vi "quiz3.5.vi"() -> ()   [LabVIEW 2017]
panel:
  out "Tab Control 2":enum32{"Login", "Menu", "Add", "delete"}(tab)
  in  "Ingresar 2":bool
  in  "Contraseña 2":string
  in  "Usuario 2":string
  in  "Delete Button 2":bool
  in  "Add Button 2":bool
  in  "Home Button 2":bool
  out "Cusuario 2":string
  in  "Previous Button 3":bool
  in  "AddContraseña 2":string
  in  "AddUsuario 2":string
  in  "Agregar 2":bool
  out "Agregado 2":bool
  in  "Cancel Button 2":bool
  in  "DeleteUsuario 2":string
  in  "Previous Button 4":bool
  out "text 2":string caption="Usuarios Activos"
  out "Tab Control":enum32{"Login", "Menu", "Add", "delete"}(tab)
  in  "Ingresar":bool
  in  "Contraseña":string
  in  "Usuario":string
  in  "Delete Button":bool
  in  "Add Button":bool
  in  "Home Button":bool
  out "Cusuario":string
  in  "Previous Button":bool
  in  "AddContraseña":string
  in  "AddUsuario":string
  in  "Agregar":bool
  out "Agregado":bool
  in  "Cancel Button":bool
  in  "DeleteUsuario":string
  in  "Previous Button 2":bool
  out "text":string caption="Usuarios Activos"
  # "USTED INGRESO CON EL USUARIO"
  # "USTED INGRESO CON EL USUARIO"
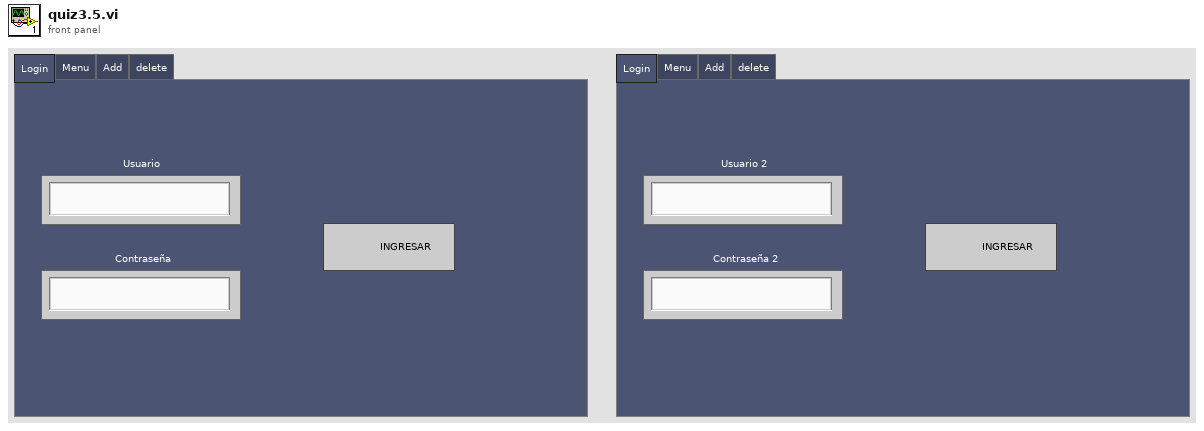
[diagram p1: front panel]
types:
  T1 = enum16{"open", "replace", "create", "open or create", "replace or create", "replace or create with confirmation"}
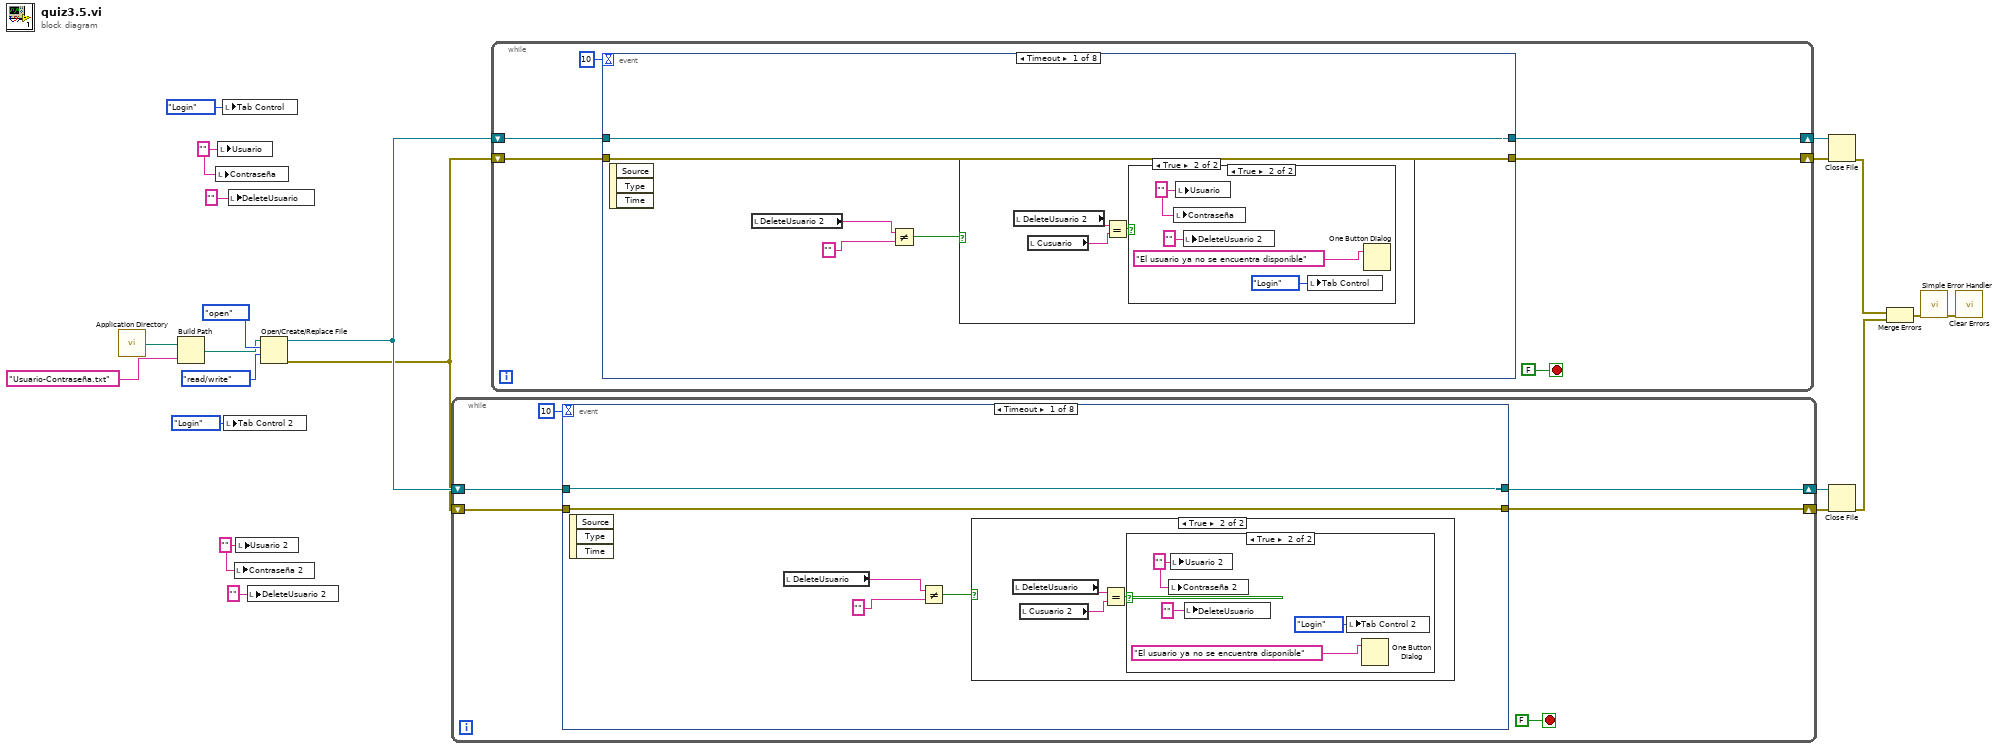
[diagram p0: block diagram]
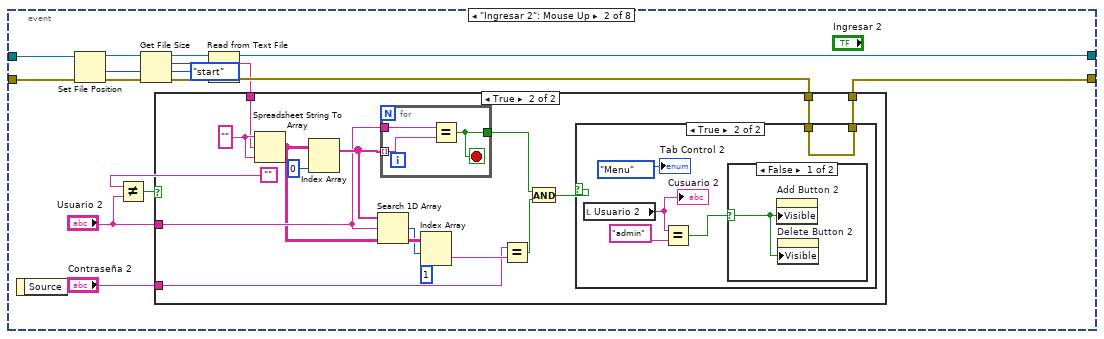
[diagram p4: hidden frame]
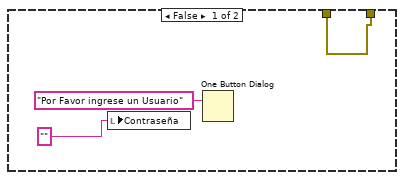
[diagram p5: hidden frame]
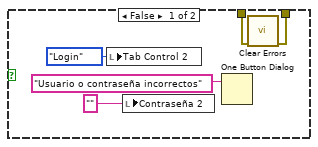
[diagram p6: hidden frame]
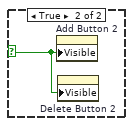
[diagram p7: hidden frame]
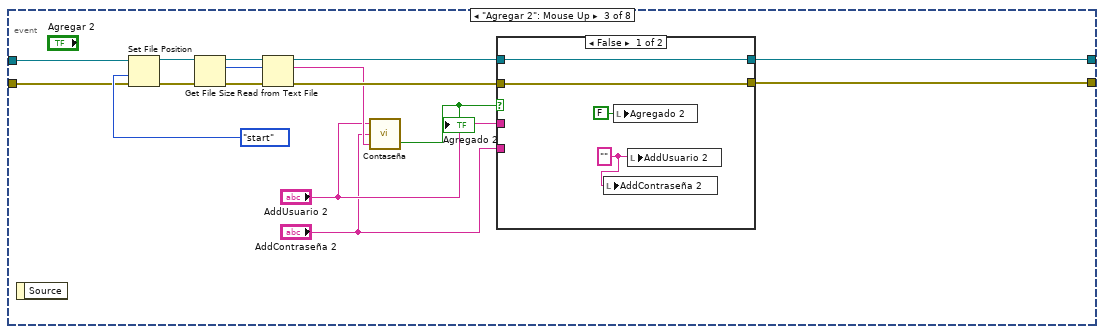
[diagram p8: hidden frame]
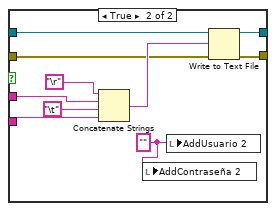
[diagram p9: hidden frame]
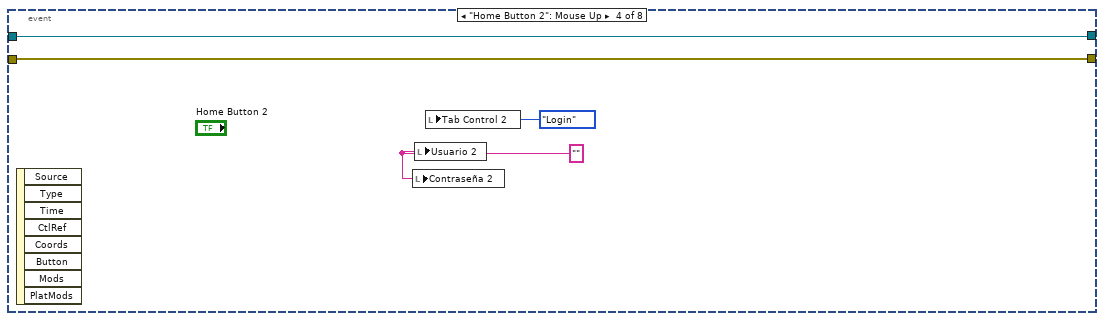
[diagram p10: hidden frame]
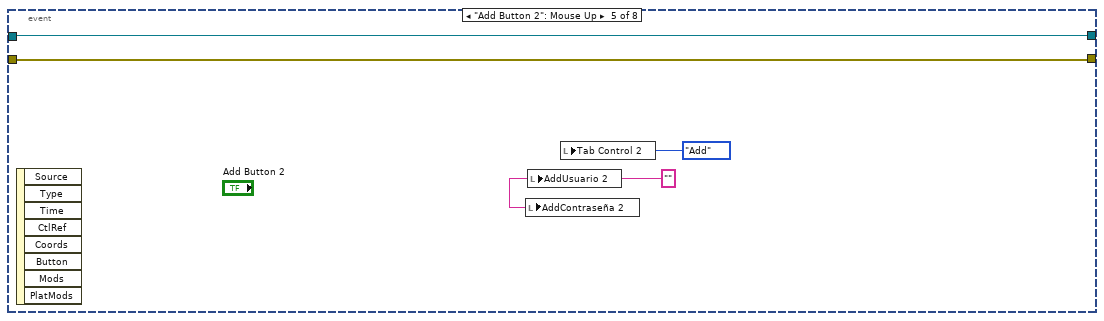
[diagram p11: hidden frame]
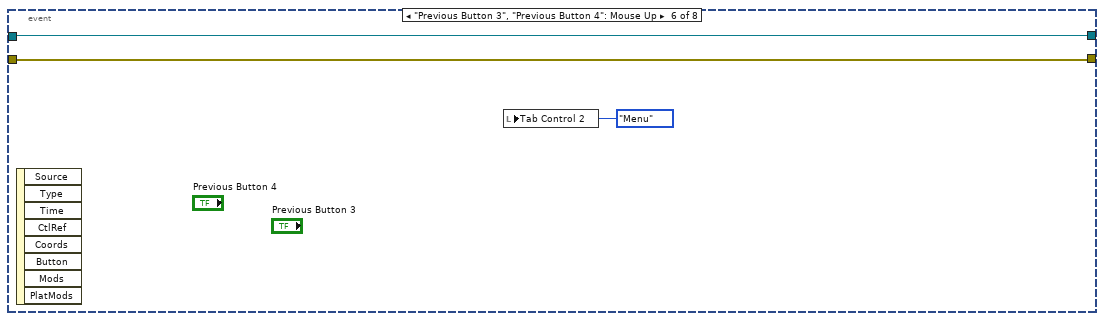
[diagram p12: hidden frame]
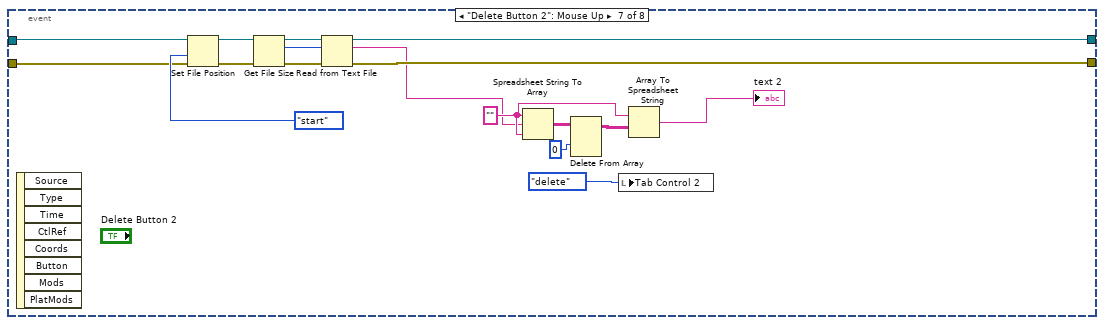
[diagram p13: hidden frame]
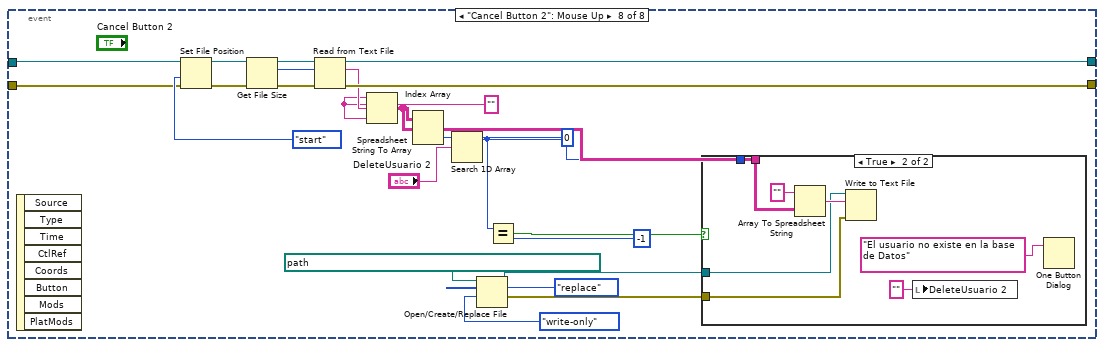
[diagram p14: hidden frame]
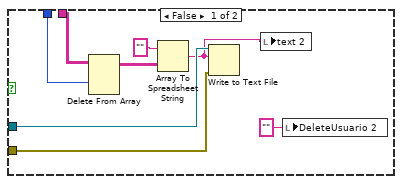
[diagram p15: hidden frame]
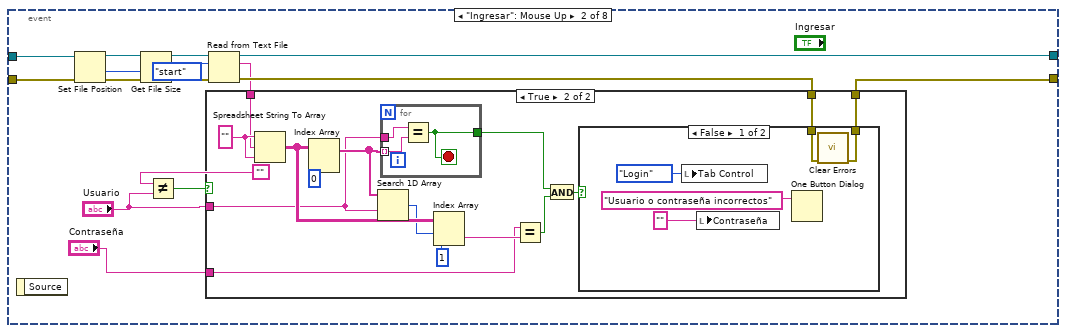
[diagram p18: hidden frame]
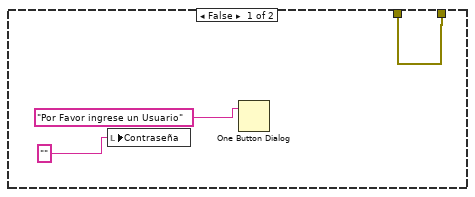
[diagram p19: hidden frame]
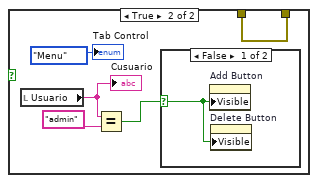
[diagram p20: hidden frame]
diagram:
  w2 = "" ("Usuario")
  w14 = "" ("Usuario")
  n1 = call <vilib>:"Application Directory.vi"() -> ("Application Directory"=w21:path)
  n2 = Build Path(base path=w21, name or relative path="Usuario-Contraseña.txt") -> (appended path=w15:path)
  n3 = local write "Contraseña"(w14) -> ()
  n4 = local write "Usuario"(w14) -> ()
  n5 = local write "Tab Control"(enum32{"Login", "Menu", "Add", "delete"}."Login" ("Tab Control")) -> ()
  n6 = local write "Tab Control 2"(enum32{"Login", "Menu", "Add", "delete"}."Login" ("Tab Control")) -> ()
  n7 = local write "DeleteUsuario"("" ("DeleteUsuario 2")) -> ()
  n8 = local write "Contraseña 2"(w2) -> ()
  n9 = local write "Usuario 2"(w2) -> ()
  n10 = local write "DeleteUsuario 2"("" ("DeleteUsuario 2")) -> ()
  n11 = Open/Create/Replace File(file path (use dialog)=w15, operation (0:open)=T1."open", access (0:read/write)=enum16{"read/write", "read-only", "write-only"}."read/write") -> (refnum out=w5:refnum<file>, error out=w3:errorcluster)  [unwired: 3 in, 1 out]
  n12 = while {
    shift-right: [w24] -> w6
    shift-left: w5 -> [w25]
    shift-right: [w23] -> w7
    shift-left: w3 -> [w26]
    stop <- FALSE stop-if-true
    n13 = event shown="[0] Timeout" {
      selector: _ -> [_ _ _ _ _ _ _ _]
      dyn-events: _ -> [_ _ _ _ _ _ _ _]
      timeout: 10 -> [_ _ _ _ _ _ _ _]
      tunnel: w26 -> [w31 w55 w92 w120 w125 w128 w137 w164]
      tunnel: [w32 w50 w104 w121 w126 w129 w138 w160] -> w24
      tunnel: [w31 w47 w103 w120 w125 w128 w136 w159] -> w23
      tunnel: w25 -> [w32 w49 w93 w121 w126 w129 w139 w163]
      event Timeout {
        n14 = event-data() -> ()  [unwired: 1 in, 3 out]
        n15 = local read "DeleteUsuario"() -> (w29:string)
        n16 = Not Equal?(x=w29, y="" ("DeleteUsuario 2")) -> (x != y?=w30:bool)
        n17 = case shown="True" w30 {
          frame False {
          }
          frame True {
            n18 = local read "DeleteUsuario"() -> (w34:string)
            n19 = local read "Cusuario 2"() -> (w33:string)
            n20 = Equal?(x=w34, y=w33) -> (x = y?=w35:bool)
            n21 = case shown="True" w35 {
              frame False {
              }
              frame True {
                w36 = "" ("Usuario")
                n22 = local write "Contraseña 2"(w36) -> ()
                n23 = local write "Usuario 2"(w36) -> ()
                n24 = local write "DeleteUsuario"("" ("DeleteUsuario 2")) -> ()
                n25 = local write "Tab Control 2"(enum32{"Login", "Menu", "Add", "delete"}."Login" ("Tab Control")) -> ()
                n26 = One Button Dialog(message="El usuario ya no se encuentra disponible") -> ()  [unwired: 1 in, 1 out]
              }
            }
          }
        }
      }
      event "Ingresar 2": Mouse Up {
        n27 = event-data() -> ()  [unwired: 1 in, 1 out]
        n28 = Set File Position(refnum=w49, from (0:start)=enum16{"start", "end", "current"}."start", error in=w55) -> (refnum out=w53:refnum<file>, error out=w54:errorcluster)  [unwired: 1 in]
        n29 = Not Equal?(x="", y="Usuario 2") -> (x != y?=w41:bool)
        n30 = Get File Size(file=w53, error in=w54) -> (refnum out=w45:refnum<file>, size (in bytes)=w52:i64, 0:w51:errorcluster)
        n31 = Read from Text File(file (use dialog)=w45, count=w52, error in=w51) -> (refnum out=w50:refnum<file>, text=w44:string, error out=w48:errorcluster)  [unwired: 1 in, 1 out]
        n32 = case shown="True" w41 {
          tunnel: w48 -> [w58 w73]
          tunnel: [w58 w72] -> w47
          tunnel: w44 -> [_ w69]
          tunnel: "Usuario 2" -> [_ w66]
          tunnel: "Contraseña 2" -> [_ w59]
          frame False {
            n33 = local write "Contraseña"("" ("Usuario")) -> ()
            n34 = One Button Dialog(message="Por Favor ingrese un Usuario") -> ()  [unwired: 1 in, 1 out]
          }
          frame True {
            w70 = "" ("format string")
            n35 = Spreadsheet String To Array(format string=w70, spreadsheet string=w69, array type (2D Dbl)=w70) -> (array=w65:string[][])  [unwired: 1 in]
            n36 = Index Array(array=w65, index (col)=0 ("index")) -> (element=w67:string[])  [unwired: 1 in]
            n37 = Search 1D Array(1D array=w67, element=w66) -> (index of element=w62:i32)  [unwired: 1 in]
            n38 = for {
              tunnel: w66 -> [w76]
              tunnel: [w75] -> w68
              tunnel: w67 -> [w74] mode=indexing
              stop <- w75 stop-if-true
              n39 = Equal?(x=w76, y=w74) -> (x = y?=w75:bool)
            }
            n40 = Index Array(array=w65, index (row)=w62, index (col)=1 ("index")) -> (element=w60:string)
            n41 = Equal?(x=w59, y=w60) -> (x = y?=w64:bool)
            n42 = And(x=w68, y=w64) -> (x .and. y?=w71:bool)
            n43 = case shown="True" w71 {
              tunnel: [w79 w86] -> w72
              tunnel: w73 -> [w78 w86]
              frame False {
                n44 = local write "Tab Control 2"(enum32{"Login", "Menu", "Add", "delete"}."Login" ("Tab Control")) -> ()
                n45 = local write "Contraseña 2"("" ("Usuario")) -> ()
                n46 = One Button Dialog(message="Usuario o contraseña incorrectos") -> ()  [unwired: 1 in, 1 out]
                n47 = call <vilib>:"Clear Errors.vi"("error in (no error)"=w78) -> ("error out"=w79:errorcluster)  [unwired: 5 in, 1 out]
              }
              frame True {
                n48 = local read "Usuario 2"() -> (w84:string)
                "Cusuario 2" <- w84
                n49 = Equal?(x=w84, y="admin") -> (x = y?=w85:bool)
                n50 = case shown="False" w85 {
                  selector: w85 -> [w87 w88]
                  frame False {
                    n51 = property on="Add Button 2" class="Bool (strict)"("Visible"=w87) -> ()  [unwired: 2 in, 2 out]
                    n52 = property on="Delete Button 2" class="Bool (strict)"("Visible"=w87) -> ()  [unwired: 2 in, 2 out]
                  }
                  frame True {
                    n53 = property on="Add Button 2" class="Bool (strict)"("Visible"=w88) -> ()  [unwired: 2 in, 2 out]
                    n54 = property on="Delete Button 2" class="Bool (strict)"("Visible"=w88) -> ()  [unwired: 2 in, 2 out]
                  }
                }
                "Tab Control 2" <- enum32{"Login", "Menu", "Add", "delete"}."Menu" ("Tab Control")
              }
            }
          }
        }
      }
      event "Agregar 2": Mouse Up {
        n55 = event-data() -> ()  [unwired: 1 in, 1 out]
        n56 = Set File Position(refnum=w93, from (0:start)=enum16{"start", "end", "current"}."start", error in=w92) -> (refnum out=w100:refnum<file>, error out=w101:errorcluster)  [unwired: 1 in]
        n57 = Get File Size(file=w100, error in=w101) -> (refnum out=w97:refnum<file>, size (in bytes)=w99:i64, 0:w98:errorcluster)
        n58 = Read from Text File(file (use dialog)=w97, count=w99, error in=w98) -> (refnum out=w95:refnum<file>, text=w91:string, error out=w94:errorcluster)  [unwired: 1 in, 1 out]
        n59 = call "Contaseña.vi"("spreadsheet string"=w91, "AddContraseña"="AddContraseña 2", "addUsuario"="AddUsuario 2") -> ("result"=w102:bool)  [unwired: 1 out]
        "Agregado 2" <- w102
        n60 = case shown="False" w102 {
          tunnel: [w108 w118] -> w104
          tunnel: [w107 w117] -> w103
          tunnel: w95 -> [w108 w113]
          tunnel: w94 -> [w107 w112]
          tunnel: "AddUsuario 2" -> [_ w111]
          tunnel: "AddContraseña 2" -> [_ w110]
          frame False {
            w106 = "" ("Usuario")
            n61 = local write "AddContraseña 2"(w106) -> ()
            n62 = local write "Agregado 2"(FALSE ("Agregado")) -> ()
            n63 = local write "AddUsuario 2"(w106) -> ()
          }
          frame True {
            w109 = "" ("Usuario")
            n64 = Concatenate Strings("\r", w111, "\t", w110) -> (w116:string)
            n65 = local write "AddContraseña 2"(w109) -> ()
            n66 = local write "AddUsuario 2"(w109) -> ()
            n67 = Write to Text File(file (use dialog)=w113, text=w116, error in=w112) -> (refnum out=w118:refnum<file>, error out=w117:errorcluster)  [unwired: 1 in, 1 out]
          }
        }
      }
      event "Home Button 2": Mouse Up {
        w122 = "" ("Usuario")
        n68 = event-data() -> ()  [unwired: 1 in, 8 out]
        n69 = local write "Contraseña 2"(w122) -> ()
        n70 = local write "Usuario 2"(w122) -> ()
        n71 = local write "Tab Control 2"(enum32{"Login", "Menu", "Add", "delete"}."Login" ("Tab Control")) -> ()
      }
      event "Add Button 2": Mouse Up {
        w123 = "" ("Usuario")
        n72 = event-data() -> ()  [unwired: 1 in, 8 out]
        n73 = local write "AddContraseña 2"(w123) -> ()
        n74 = local write "AddUsuario 2"(w123) -> ()
        n75 = local write "Tab Control 2"(enum32{"Login", "Menu", "Add", "delete"}."Add" ("Tab Control")) -> ()
      }
      event "Previous Button 3", "Previous Button 4": Mouse Up {
        n76 = event-data() -> ()  [unwired: 1 in, 8 out]
        n77 = local write "Tab Control 2"(enum32{"Login", "Menu", "Add", "delete"}."Menu" ("Tab Control")) -> ()
      }
      event "Delete Button 2": Mouse Up {
        w135 = "" ("format string")
        n78 = event-data() -> ()  [unwired: 1 in, 8 out]
        n79 = Set File Position(refnum=w139, from (0:start)=enum16{"start", "end", "current"}."start", error in=w137) -> (refnum out=w144:refnum<file>, error out=w145:errorcluster)  [unwired: 1 in]
        n80 = Get File Size(file=w144, error in=w145) -> (refnum out=w141:refnum<file>, size (in bytes)=w143:i64, 0:w142:errorcluster)
        n81 = Read from Text File(file (use dialog)=w141, count=w143, error in=w142) -> (refnum out=w138:refnum<file>, text=w131:string, error out=w136:errorcluster)  [unwired: 1 in, 1 out]
        n82 = Spreadsheet String To Array(format string=w135, spreadsheet string=w131, array type (2D Dbl)=w135) -> (array=w133:string[][])  [unwired: 1 in]
        n83 = Delete From Array(array=w133, index (row)=0) -> (array with subset deleted=w132:string[][])  [unwired: 2 in, 1 out]
        n84 = local write "Tab Control 2"(enum32{"Login", "Menu", "Add", "delete"}."delete" ("Tab Control")) -> ()
        n85 = Array To Spreadsheet String(array=w132, 3:w135) -> (spreadsheet string=→"text 2":string)  [unwired: 1 in]
      }
      event "Cancel Button 2": Mouse Up {
        w156 = "" ("format string")
        n86 = event-data() -> ()  [unwired: 1 in, 8 out]
        n87 = Set File Position(refnum=w163, from (0:start)=enum16{"start", "end", "current"}."start", error in=w164) -> (refnum out=w169:refnum<file>, error out=w170:errorcluster)  [unwired: 1 in]
        n88 = Get File Size(file=w169, error in=w170) -> (refnum out=w166:refnum<file>, size (in bytes)=w168:i64, 0:w167:errorcluster)
        n89 = Read from Text File(file (use dialog)=w166, count=w168, error in=w167) -> (refnum out=w160:refnum<file>, text=w157:string, error out=w159:errorcluster)  [unwired: 1 in, 1 out]
        n90 = Spreadsheet String To Array(format string=w156, spreadsheet string=w157, array type (2D Dbl)=w156) -> (array=w152:string[][])  [unwired: 1 in]
        n91 = Index Array(array=w152, index (col)=0 ("disabled index (col)")) -> (element=w154:string[])  [unwired: 1 in]
        n92 = Search 1D Array(1D array=w154, element="DeleteUsuario 2") -> (index of element=w148:i32)  [unwired: 1 in]
        n93 = Open/Create/Replace File(file path (use dialog)=path "D:/2019-1/Programacion 2/quiz 3/Usuario-Contraseña.txt", operation (0:open)=T1."replace", access (0:read/write)=enum16{"read/write", "read-only", "write-only"}."write-only") -> (refnum out=w151:refnum<file>, error out=w150:errorcluster)  [unwired: 3 in, 1 out]
        n94 = Equal?(x=w148, y=-1) -> (x = y?=w149:bool)
        n95 = case shown="True" w149 {
          tunnel: w152 -> [w178 w181]
          tunnel: w148 -> [w177 _]
          tunnel: w151 -> [w175 w180]
          tunnel: w150 -> [w174 w179]
          frame False {
            n96 = Delete From Array(array=w178, index (row)=w177) -> (array with subset deleted=w176:string[][])  [unwired: 2 in, 1 out]
            n97 = Array To Spreadsheet String(array=w176, 3:"" ("format string")) -> (spreadsheet string=w172:string)  [unwired: 1 in]
            n98 = Write to Text File(file (use dialog)=w175, text=w172, error in=w174) -> ()  [unwired: 1 in, 3 out]
            n99 = local write "text 2"(w172) -> ()
            n100 = local write "DeleteUsuario 2"("" ("DeleteUsuario 2")) -> ()
          }
          frame True {
            n101 = Array To Spreadsheet String(array=w181, 3:"" ("format string")) -> (spreadsheet string=w183:string)  [unwired: 1 in]
            n102 = Write to Text File(file (use dialog)=w180, text=w183, error in=w179) -> ()  [unwired: 1 in, 3 out]
            n103 = local write "DeleteUsuario 2"("" ("DeleteUsuario 2")) -> ()
            n104 = One Button Dialog(message="El usuario no existe en la base de Datos") -> ()  [unwired: 1 in, 1 out]
          }
        }
      }
    }
  }
  n105 = while {
    shift-right: [w188] -> w11
    shift-left: w5 -> [w189]
    shift-right: [w187] -> w16
    shift-left: w3 -> [w190]
    stop <- FALSE stop-if-true
    n106 = event shown="[0] Timeout" {
      selector: _ -> [_ _ _ _ _ _ _ _]
      dyn-events: _ -> [_ _ _ _ _ _ _ _]
      timeout: 10 -> [_ _ _ _ _ _ _ _]
      tunnel: w190 -> [w195 w219 w257 w284 w289 w292 w301 w328]
      tunnel: [w196 w214 w268 w285 w290 w293 w302 w324] -> w188
      tunnel: [w195 w211 w253 w284 w289 w292 w300 w323] -> w187
      tunnel: w189 -> [w196 w213 w258 w285 w290 w293 w303 w327]
      event Timeout {
        n107 = event-data() -> ()  [unwired: 1 in, 3 out]
        n108 = local read "DeleteUsuario 2"() -> (w193:string)
        n109 = Not Equal?(x=w193, y="" ("DeleteUsuario 2")) -> (x != y?=w192:bool)
        n110 = case shown="True" w192 {
          frame False {
          }
          frame True {
            n111 = local read "DeleteUsuario 2"() -> (w197:string)
            n112 = local read "Cusuario"() -> (w198:string)
            n113 = Equal?(x=w197, y=w198) -> (x = y?=w199:bool)
            n114 = case shown="True" w199 {
              frame False {
              }
              frame True {
                w200 = "" ("Usuario")
                n115 = local write "Contraseña"(w200) -> ()
                n116 = local write "Usuario"(w200) -> ()
                n117 = local write "DeleteUsuario 2"("" ("DeleteUsuario 2")) -> ()
                n118 = local write "Tab Control"(enum32{"Login", "Menu", "Add", "delete"}."Login" ("Tab Control")) -> ()
                n119 = One Button Dialog(message="El usuario ya no se encuentra disponible") -> ()  [unwired: 1 in, 1 out]
              }
            }
          }
        }
      }
      event "Ingresar": Mouse Up {
        n120 = event-data() -> ()  [unwired: 1 in, 1 out]
        n121 = Set File Position(refnum=w213, from (0:start)=enum16{"start", "end", "current"}."start", error in=w219) -> (refnum out=w217:refnum<file>, error out=w218:errorcluster)  [unwired: 1 in]
        n122 = Get File Size(file=w217, error in=w218) -> (refnum out=w209:refnum<file>, size (in bytes)=w216:i64, 0:w215:errorcluster)
        n123 = Not Equal?(x="", y="Usuario") -> (x != y?=w206:bool)
        n124 = Read from Text File(file (use dialog)=w209, count=w216, error in=w215) -> (refnum out=w214:refnum<file>, text=w208:string, error out=w212:errorcluster)  [unwired: 1 in, 1 out]
        n125 = case shown="True" w206 {
          tunnel: w212 -> [w222 w237]
          tunnel: [w222 w236] -> w211
          tunnel: w208 -> [_ w233]
          tunnel: "Usuario" -> [_ w224]
          tunnel: "Contraseña" -> [_ w223]
          frame False {
            n126 = local write "Contraseña"("" ("Usuario")) -> ()
            n127 = One Button Dialog(message="Por Favor ingrese un Usuario") -> ()  [unwired: 1 in, 1 out]
          }
          frame True {
            w234 = "" ("format string")
            n128 = Spreadsheet String To Array(format string=w234, spreadsheet string=w233, array type (2D Dbl)=w234) -> (array=w230:string[][])  [unwired: 1 in]
            n129 = Index Array(array=w230, index (col)=0 ("index")) -> (element=w231:string[])  [unwired: 1 in]
            n130 = Search 1D Array(1D array=w231, element=w224) -> (index of element=w227:i32)  [unwired: 1 in]
            n131 = for {
              tunnel: [w240] -> w232
              tunnel: w231 -> [w239] mode=indexing
              tunnel: w224 -> [w238]
              stop <- w240 stop-if-true
              n132 = Equal?(x=w238, y=w239) -> (x = y?=w240:bool)
            }
            n133 = Index Array(array=w230, index (row)=w227, index (col)=1 ("index")) -> (element=w225:string)
            n134 = Equal?(x=w223, y=w225) -> (x = y?=w229:bool)
            n135 = And(x=w232, y=w229) -> (x .and. y?=w235:bool)
            n136 = case shown="False" w235 {
              tunnel: [w243 w250] -> w236
              tunnel: w237 -> [w242 w250]
              frame False {
                n137 = local write "Tab Control"(enum32{"Login", "Menu", "Add", "delete"}."Login" ("Tab Control")) -> ()
                n138 = local write "Contraseña"("" ("Usuario")) -> ()
                n139 = One Button Dialog(message="Usuario o contraseña incorrectos") -> ()  [unwired: 1 in, 1 out]
                n140 = call <vilib>:"Clear Errors.vi"("error in (no error)"=w242) -> ("error out"=w243:errorcluster)  [unwired: 5 in, 1 out]
              }
              frame True {
                n141 = local read "Usuario"() -> (w248:string)
                "Cusuario" <- w248
                n142 = Equal?(x=w248, y="admin") -> (x = y?=w249:bool)
                n143 = case shown="False" w249 {
                  selector: w249 -> [w251 w252]
                  frame False {
                    n144 = property on="Add Button" class="Bool (strict)"("Visible"=w251) -> ()  [unwired: 2 in, 2 out]
                    n145 = property on="Delete Button" class="Bool (strict)"("Visible"=w251) -> ()  [unwired: 2 in, 2 out]
                  }
                  frame True {
                    n146 = property on="Add Button" class="Bool (strict)"("Visible"=w252) -> ()  [unwired: 2 in, 2 out]
                    n147 = property on="Delete Button" class="Bool (strict)"("Visible"=w252) -> ()  [unwired: 2 in, 2 out]
                  }
                }
                "Tab Control" <- enum32{"Login", "Menu", "Add", "delete"}."Menu" ("Tab Control")
              }
            }
          }
        }
      }
      event "Agregar": Mouse Up {
        n148 = event-data() -> ()  [unwired: 1 in, 1 out]
        n149 = Set File Position(refnum=w258, from (0:start)=enum16{"start", "end", "current"}."start", error in=w257) -> (refnum out=w265:refnum<file>, error out=w266:errorcluster)  [unwired: 1 in]
        n150 = Get File Size(file=w265, error in=w266) -> (refnum out=w262:refnum<file>, size (in bytes)=w264:i64, 0:w263:errorcluster)
        n151 = Read from Text File(file (use dialog)=w262, count=w264, error in=w263) -> (refnum out=w260:refnum<file>, text=w256:string, error out=w259:errorcluster)  [unwired: 1 in, 1 out]
        n152 = call "Contaseña.vi"("spreadsheet string"=w256, "AddContraseña"="AddContraseña", "addUsuario"="AddUsuario") -> ("result"=w267:bool)  [unwired: 1 out]
        "Agregado" <- w267
        n153 = case shown="False" w267 {
          tunnel: [w272 w282] -> w268
          tunnel: [w271 w281] -> w253
          tunnel: w260 -> [w272 w277]
          tunnel: w259 -> [w271 w276]
          tunnel: "AddUsuario" -> [_ w275]
          tunnel: "AddContraseña" -> [_ w274]
          frame False {
            w270 = "" ("Usuario")
            n154 = local write "AddContraseña"(w270) -> ()
            n155 = local write "Agregado"(FALSE ("Agregado")) -> ()
            n156 = local write "AddUsuario"(w270) -> ()
          }
          frame True {
            w273 = "" ("Usuario")
            n157 = Concatenate Strings("\r", w275, "\t", w274) -> (w280:string)
            n158 = local write "AddContraseña"(w273) -> ()
            n159 = local write "AddUsuario"(w273) -> ()
            n160 = Write to Text File(file (use dialog)=w277, text=w280, error in=w276) -> (refnum out=w282:refnum<file>, error out=w281:errorcluster)  [unwired: 1 in, 1 out]
          }
        }
      }
      event "Home Button": Mouse Up {
        w286 = "" ("Usuario")
        n161 = event-data() -> ()  [unwired: 1 in, 8 out]
        n162 = local write "Contraseña"(w286) -> ()
        n163 = local write "Usuario"(w286) -> ()
        n164 = local write "Tab Control"(enum32{"Login", "Menu", "Add", "delete"}."Login" ("Tab Control")) -> ()
      }
      event "Add Button": Mouse Up {
        w288 = "" ("Usuario")
        n165 = event-data() -> ()  [unwired: 1 in, 8 out]
        n166 = local write "AddContraseña"(w288) -> ()
        n167 = local write "AddUsuario"(w288) -> ()
        n168 = local write "Tab Control"(enum32{"Login", "Menu", "Add", "delete"}."Add" ("Tab Control")) -> ()
      }
      event "Previous Button", "Previous Button 2": Mouse Up {
        n169 = event-data() -> ()  [unwired: 1 in, 8 out]
        n170 = local write "Tab Control"(enum32{"Login", "Menu", "Add", "delete"}."Menu" ("Tab Control")) -> ()
      }
      event "Delete Button": Mouse Up {
        w296 = "" ("format string")
        n171 = event-data() -> ()  [unwired: 1 in, 8 out]
        n172 = Set File Position(refnum=w303, from (0:start)=enum16{"start", "end", "current"}."start", error in=w301) -> (refnum out=w308:refnum<file>, error out=w309:errorcluster)  [unwired: 1 in]
        n173 = Get File Size(file=w308, error in=w309) -> (refnum out=w305:refnum<file>, size (in bytes)=w307:i64, 0:w306:errorcluster)
        n174 = Read from Text File(file (use dialog)=w305, count=w307, error in=w306) -> (refnum out=w302:refnum<file>, text=w294:string, error out=w300:errorcluster)  [unwired: 1 in, 1 out]
        n175 = local write "Tab Control"(enum32{"Login", "Menu", "Add", "delete"}."delete" ("Tab Control")) -> ()
        n176 = Spreadsheet String To Array(format string=w296, spreadsheet string=w294, array type (2D Dbl)=w296) -> (array=w298:string[][])  [unwired: 1 in]
        n177 = Delete From Array(array=w298, index (row)=0) -> (array with subset deleted=w299:string[][])  [unwired: 2 in, 1 out]
        n178 = Array To Spreadsheet String(array=w299, 3:w296) -> (spreadsheet string=→"text":string)  [unwired: 1 in]
      }
      event "Cancel Button": Mouse Up {
        w320 = "" ("format string")
        n179 = event-data() -> ()  [unwired: 1 in, 8 out]
        n180 = Set File Position(refnum=w327, from (0:start)=enum16{"start", "end", "current"}."start", error in=w328) -> (refnum out=w333:refnum<file>, error out=w334:errorcluster)  [unwired: 1 in]
        n181 = Get File Size(file=w333, error in=w334) -> (refnum out=w330:refnum<file>, size (in bytes)=w332:i64, 0:w331:errorcluster)
        n182 = Read from Text File(file (use dialog)=w330, count=w332, error in=w331) -> (refnum out=w324:refnum<file>, text=w321:string, error out=w323:errorcluster)  [unwired: 1 in, 1 out]
        n183 = Spreadsheet String To Array(format string=w320, spreadsheet string=w321, array type (2D Dbl)=w320) -> (array=w316:string[][])  [unwired: 1 in]
        n184 = Index Array(array=w316, index (col)=0 ("disabled index (col)")) -> (element=w318:string[])  [unwired: 1 in]
        n185 = Search 1D Array(1D array=w318, element="DeleteUsuario") -> (index of element=w312:i32)  [unwired: 1 in]
        n186 = Open/Create/Replace File(file path (use dialog)=path "D:/2019-1/Programacion 2/quiz 3/Usuario-Contraseña.txt", operation (0:open)=T1."replace", access (0:read/write)=enum16{"read/write", "read-only", "write-only"}."write-only") -> (refnum out=w315:refnum<file>, error out=w314:errorcluster)  [unwired: 3 in, 1 out]
        n187 = Equal?(x=w312, y=-1) -> (x = y?=w313:bool)
        n188 = case shown="False" w313 {
          tunnel: w316 -> [w342 w345]
          tunnel: w312 -> [w341 _]
          tunnel: w315 -> [w339 w344]
          tunnel: w314 -> [w338 w343]
          frame False {
            n189 = Delete From Array(array=w342, index (row)=w341) -> (array with subset deleted=w340:string[][])  [unwired: 2 in, 1 out]
            n190 = Array To Spreadsheet String(array=w340, 3:"" ("format string")) -> (spreadsheet string=w336:string)  [unwired: 1 in]
            n191 = Write to Text File(file (use dialog)=w339, text=w336, error in=w338) -> ()  [unwired: 1 in, 3 out]
            n192 = local write "text"(w336) -> ()
            n193 = local write "DeleteUsuario"("" ("DeleteUsuario 2")) -> ()
          }
          frame True {
            n194 = Array To Spreadsheet String(array=w345, 3:"" ("format string")) -> (spreadsheet string=w347:string)  [unwired: 1 in]
            n195 = Write to Text File(file (use dialog)=w344, text=w347, error in=w343) -> ()  [unwired: 1 in, 3 out]
            n196 = local write "DeleteUsuario"("" ("DeleteUsuario 2")) -> ()
            n197 = One Button Dialog(message="El usuario no existe en la base de Datos") -> ()  [unwired: 1 in, 1 out]
          }
        }
      }
    }
  }
  n198 = Close File(refnum=w11, error in=w16) -> (error out=w9:errorcluster)  [unwired: 1 out]
  n199 = Close File(refnum=w6, error in=w7) -> (error out=w8:errorcluster)  [unwired: 1 out]
  n200 = Merge Errors(w9, w8) -> (w10:errorcluster)
  n201 = call <vilib>:"Simple Error Handler.vi"("error in (no error)"=w10) -> ("error out"=w17:errorcluster)  [unwired: 4 in, 4 out]
  n202 = call <vilib>:"Clear Errors.vi"("error in (no error)"=w17) -> ()  [unwired: 5 in, 2 out]
